vi "음료자판기.vi"(10 "구매":bool, 11 "음료":u8(knob) max=2 step=1 scale=0.0..2.0) -> ()   [LabVIEW 2014]
panel:
  in  "음료수량 초기값":cluster{"콜라":u8, "사이다":u8, "생수":u8}={"콜라"=10, "사이다"=10, "생수"=10}
  in  "정지":bool
  out "생수":u8
  out "사이다":u8
  out "콜라":u8
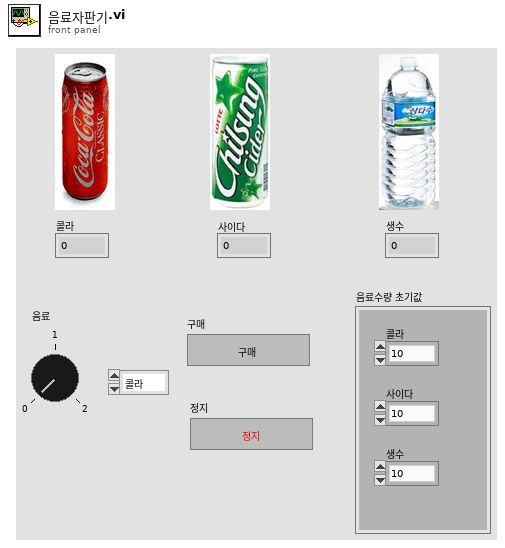
[diagram p1: front panel]
types:
  T1 = typedef "음료.ctl" = enum16{"초기화", "Idle", "구매", "음료확인", "정지"}
  T2 = enum8{"Enabled", "Disabled", "Disabled and Grayed Out"}
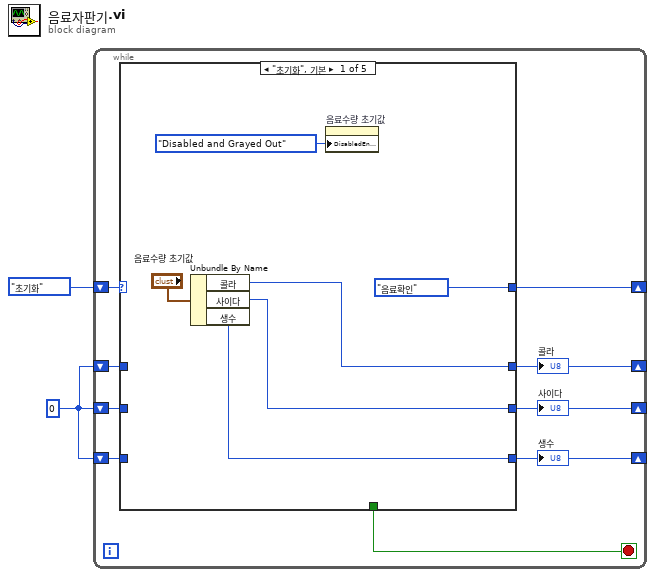
[diagram p0: block diagram]
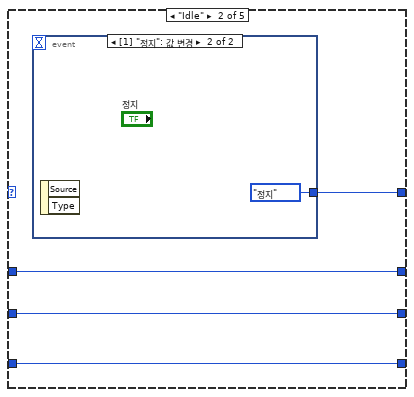
[diagram p2: hidden frame]
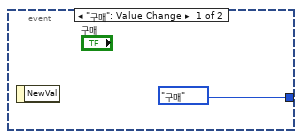
[diagram p3: hidden frame]
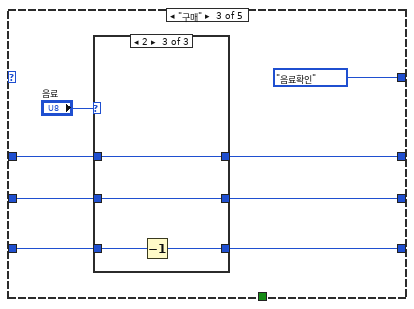
[diagram p4: hidden frame]
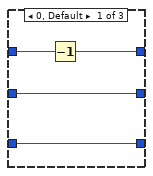
[diagram p5: hidden frame]
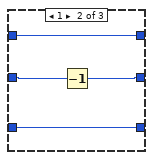
[diagram p6: hidden frame]
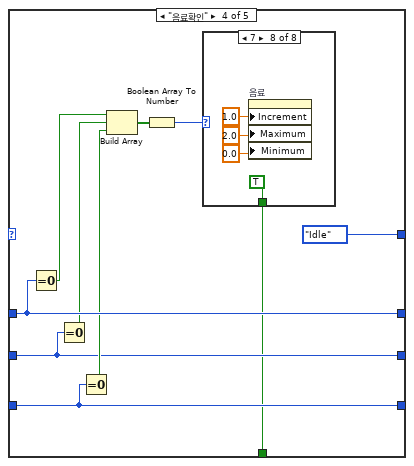
[diagram p7: hidden frame]
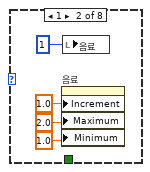
[diagram p9: hidden frame]
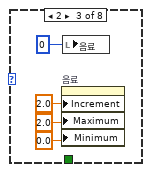
[diagram p10: hidden frame]
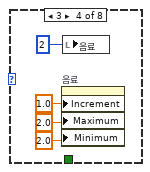
[diagram p11: hidden frame]
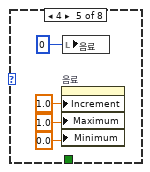
[diagram p12: hidden frame]
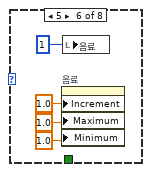
[diagram p13: hidden frame]
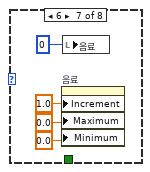
[diagram p14: hidden frame]
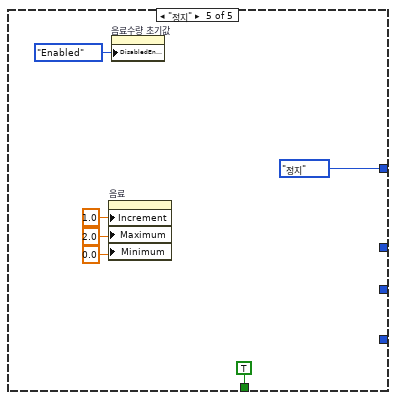
[diagram p15: hidden frame]
diagram:
  w1 = u8 0 ("콜라")
  n1 = while {
    shift-right: [w10] -> _
    shift-left: 음료."초기화" ("열거형") -> [w11]
    shift-right: [w7] -> _
    shift-left: w1 -> [w6]
    shift-right: [w8] -> _
    shift-left: w1 -> [w5]
    shift-right: [w9] -> _
    shift-left: w1 -> [w4]
    stop <- w3 stop-if-true
    n2 = case shown="\"초기화\", 기본" w11 {
      tunnel: [w16 w21 w28 w52 _] -> w7
      tunnel: [w15 w20 w26 w47 _] -> w8
      tunnel: [w14 w19 w24 w46 _] -> w9
      tunnel: [음료."음료확인" ("열거형") w18 음료."음료확인" ("열거형") 음료."Idle" ("열거형") 음료."정지" ("열거형")] -> w10
      tunnel: w6 -> [_ w21 w29 w52 _]
      tunnel: w5 -> [_ w20 w27 w47 _]
      tunnel: w4 -> [_ w19 w25 w46 _]
      tunnel: [_ _ _ w44 TRUE] -> w3
      frame "초기화", Default {
        n3 = Unbundle By Name("음료수량 초기값") -> ("콜라"=w16:u8, "사이다"=w15:u8, "생수"=w14:u8)
        n4 = property on="음료수량 초기값" class="Clust (엄격한)"("DisabledEnum"=T2."Disabled and Grayed Out" ("비활성화")) -> ()  [unwired: 2 in, 2 out]
      }
      frame "Idle" {
        n5 = event shown="[1] \"정지\": 값 변경" {
          selector: _ -> [_ _]
          dyn-events: _ -> [_ _]
          timeout: _ -> [_ _]
          tunnel: [음료."구매" ("열거형") 음료."정지" ("열거형")] -> w18
          event "구매": Value Change {
            n6 = event-data() -> ()  [unwired: 1 in, 1 out]
          }
          event "정지": Value Change {
            n7 = event-data() -> ()  [unwired: 1 in, 2 out]
          }
        }
      }
      frame "구매" {
        n8 = case shown="2" "음료" {
          tunnel: w29 -> [w35 w39 w43]
          tunnel: [w34 w39 w43] -> w28
          tunnel: w27 -> [w33 w38 w42]
          tunnel: [w33 w37 w42] -> w26
          tunnel: w25 -> [w32 w36 w41]
          tunnel: [w32 w36 w40] -> w24
          frame 0, Default {
            n9 = Decrement(x=w35) -> (x-1=w34:u8)
          }
          frame 1 {
            n10 = Decrement(x=w38) -> (x-1=w37:u8)
          }
          frame 2 {
            n11 = Decrement(x=w41) -> (x-1=w40:u8)
          }
        }
      }
      frame "음료확인" {
        n12 = Equal To 0?(x=w52) -> (x = 0?=w51:bool)
        n13 = Equal To 0?(x=w47) -> (x = 0?=w50:bool)
        n14 = Equal To 0?(x=w46) -> (x = 0?=w49:bool)
        n15 = Build Array(w51, w50, w49) -> (w48:bool[])
        n16 = Boolean Array To Number(Boolean array=w48) -> (number=w45:u32)
        n17 = case shown="7" w45 {
          tunnel: [_ _ _ _ _ _ _ TRUE] -> w44
          frame 0, Default {
          }
          frame 1 {
            n18 = property on="음료" class="Knob (엄격한)"("Increment"=1.0 ("데이터 입력 제한:증가"), "Maximum"=2.0 ("데이터 입력 제한:최대"), "Minimum"=1.0 ("데이터 입력 제한:최소")) -> ()  [unwired: 2 in, 2 out]
            n19 = local write "음료"(u8 1) -> ()
          }
          frame 2 {
            n20 = property on="음료" class="Knob (엄격한)"("Increment"=2.0 ("데이터 입력 제한:증가"), "Maximum"=2.0 ("데이터 입력 제한:최대"), "Minimum"=0.0 ("데이터 입력 제한:최소")) -> ()  [unwired: 2 in, 2 out]
            n21 = local write "음료"(u8 0) -> ()
          }
          frame 3 {
            n22 = property on="음료" class="Knob (엄격한)"("Increment"=1.0 ("데이터 입력 제한:증가"), "Maximum"=2.0 ("데이터 입력 제한:최대"), "Minimum"=2.0 ("데이터 입력 제한:최소")) -> ()  [unwired: 2 in, 2 out]
            n23 = local write "음료"(u8 2) -> ()
          }
          frame 4 {
            n24 = property on="음료" class="Knob (엄격한)"("Increment"=1.0 ("데이터 입력 제한:증가"), "Maximum"=1.0 ("데이터 입력 제한:최대"), "Minimum"=0.0 ("데이터 입력 제한:최소")) -> ()  [unwired: 2 in, 2 out]
            n25 = local write "음료"(u8 0) -> ()
          }
          frame 5 {
            n26 = property on="음료" class="Knob (엄격한)"("Increment"=1.0 ("데이터 입력 제한:증가"), "Maximum"=1.0 ("데이터 입력 제한:최대"), "Minimum"=1.0 ("데이터 입력 제한:최소")) -> ()  [unwired: 2 in, 2 out]
            n27 = local write "음료"(u8 1) -> ()
          }
          frame 6 {
            n28 = property on="음료" class="Knob (엄격한)"("Increment"=1.0 ("데이터 입력 제한:증가"), "Maximum"=0.0 ("데이터 입력 제한:최대"), "Minimum"=0.0 ("데이터 입력 제한:최소")) -> ()  [unwired: 2 in, 2 out]
            n29 = local write "음료"(u8 0) -> ()
          }
          frame 7 {
            n30 = property on="음료" class="Knob (엄격한)"("Increment"=1.0 ("데이터 입력 제한:증가"), "Maximum"=2.0 ("데이터 입력 제한:최대"), "Minimum"=0.0 ("데이터 입력 제한:최소")) -> ()  [unwired: 2 in, 2 out]
          }
        }
      }
      frame "정지" {
        n31 = property on="음료" class="Knob (엄격한)"("Increment"=1.0 ("데이터 입력 제한:증가"), "Maximum"=2.0 ("데이터 입력 제한:최대"), "Minimum"=0.0 ("데이터 입력 제한:최소")) -> ()  [unwired: 2 in, 2 out]
        n32 = property on="음료수량 초기값" class="Clust (엄격한)"("DisabledEnum"=T2."Enabled" ("비활성화")) -> ()  [unwired: 2 in, 2 out]
      }
    }
    "생수" <- w9
    "사이다" <- w8
    "콜라" <- w7
  }
